vi "xy_bar_graph.vi"() -> ()   [LabVIEW 2016]
doc: "This VI demonstrates how to create a bar graph in LabVIEW by plotting data to an XY graph. This VI converts the data that appears in a table to bars and groups the bars by column of data from the table."
panel:
  out "Annual Report":cluster{dbl[], dbl[]}[](graph)
  in  "Table":string[][](table)=[["34", "74", "23", "35", "23", "26", "74", "74", "21", "39", "61", "83"], ["73", "24", "75", "87", "42", "34", "35", "76", "52", "43", "43", "3"], ["36", "25", "12", "34", "24", "74", "73", "54", "88", "64", "90", "62"]]
  # "This VI graphs the data from the Table to the Annual Report graph.  Select Help»Show Context Help and move the cursor over the VI icon to display help for this VI."
  # "Jan"
  # "Feb"
  # "Mar"
  # "April"
  # "May"
  # "June"
  # "July"
  # "Aug"
  # "Sept"
  # "Oct"
  # "Nov"
  # "Dec"
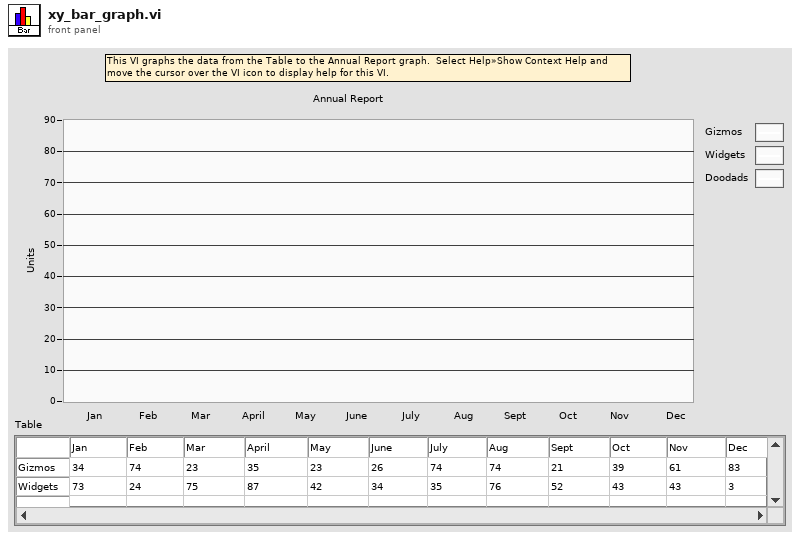
[diagram p1: front panel]
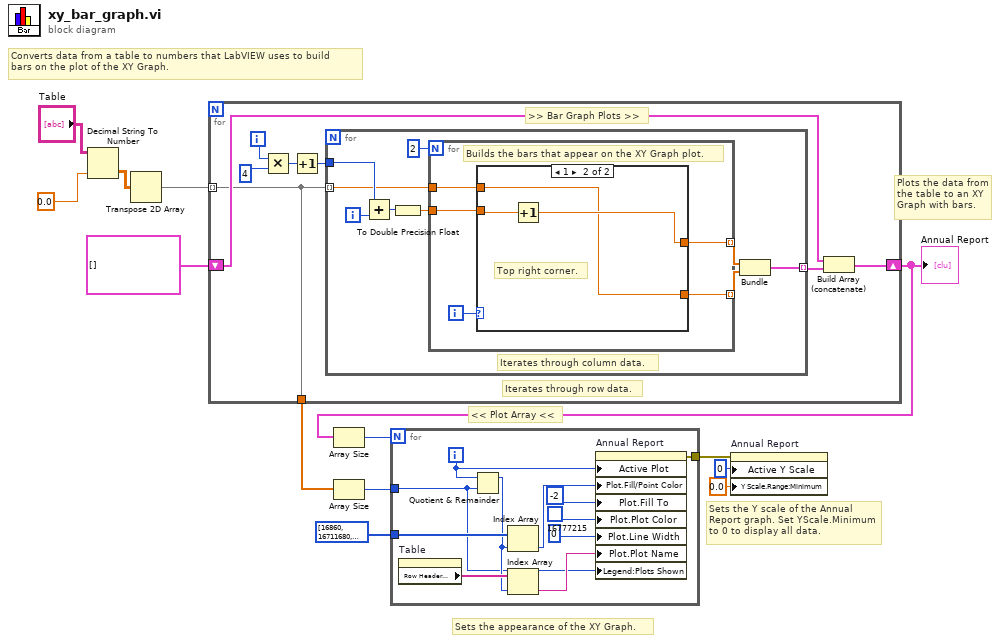
[diagram p0: block diagram]
diagram:
  # "Plots the data from the table to an XY Graph with bars."
  # "Converts data from a table to numbers that LabVIEW uses to build \nbars on the plot of the XY Graph."
  # "Sets the appearance of the XY Graph."
  # "Sets the Y scale of the Annual Report graph. Set YScale.Minimum to 0 to display all data."
  # "<< Plot Array <<"
  n1 = Decimal String To Number(string="Table", default (0L)=0.0) -> (number=w11:dbl[][])  [unwired: 1 in, 1 out]
  n2 = Transpose 2D Array(2D array=w11) -> (transposed array=w10:dbl[][])
  n3 = for {
    tunnel: w10 -> [w14] mode=indexing
    shift-right: [w18] -> w8
    shift-left: cluster{dbl[], dbl[]}[] [] -> [w17]
    tunnel: [w14] -> w6
    i -> [w21]
    # "Iterates through row data."
    # ">> Bar Graph Plots >>"
    n4 = Multiply(x=w21, y=4) -> (x*y=w16:i32)
    n5 = Increment(x=w16) -> (x+1=w15:i32)
    n6 = for {
      tunnel: w14 -> [w23] mode=indexing
      tunnel: w15 -> [w30]
      tunnel: [w25] -> w19 mode=indexing
      i -> [w24]
      # "Iterates through column data."
      n7 = Add(x=w30, y=w24) -> (x+y=w29:i32)
      n8 = To Double Precision Float(number=w29) -> (double precision float=w28:dbl)
      n9 = for {
        N: 2 -> [_]
        tunnel: w23 -> [w34]
        tunnel: [w33] -> w26 mode=indexing
        tunnel: w28 -> [w32]
        tunnel: [w31] -> w27 mode=indexing
        i -> [w35]
        # "Builds the bars that appear on the XY Graph plot."
        n10 = case shown="1" w35 {
          tunnel: w34 -> [w37 w38]
          tunnel: [w37 w38] -> w33
          tunnel: w32 -> [w36 w40]
          tunnel: [w36 w39] -> w31
          frame 0, Default {
            # "Top left corner."
          }
          frame 1 {
            # "Top right corner."
            n11 = Increment(x=w40) -> (x+1=w39:dbl)
          }
        }
      }
      n12 = Bundle(w27, w26) -> (w25:cluster{dbl[], dbl[]})  [unwired: 1 in]
    }
    n13 = Build Array (concatenate) "Build Array"(w17, w19) -> (w18:cluster{dbl[], dbl[]}[])
  }
  "Annual Report" <- w8
  n14 = Array Size(array=w8) -> (size(s)=w7:i32)
  n15 = Array Size(array=w6) -> (size(s)=w5:i32)
  n16 = for {
    N: w7 -> [_]
    tunnel: w5 -> [w42]
    tunnel: u32[] [16860, 16711680, 1175296, 16773632, 15679744, 16711925, 2818015, 4325415] -> [w47]
    tunnel: [w41] -> w3
    i -> [w51]
    n17 = property on="Table" class="Tbl (strict)"() -> ("Row Header Strings[]"=w45:string[])  [unwired: 2 in, 2 out]
    n18 = Quotient & Remainder(x=w51, y=w42) -> (x-y*floor(x/y)=w44:i32)  [unwired: 1 out]
    n19 = Index Array(array=w47, index=w44) -> (element=w50:u32)
    n20 = Index Array(array=w45, index=w44) -> (element=w43:string)
    n21 = property on="Annual Report" class="XYGraph (strict)"("Active Plot"=w51, "Plot.Fill/Point Color"=w50, "Plot.Fill To"=i16 -2, "Plot.Plot Color"=u32 16777215, "Plot.Line Width"=u8 0, "Plot.Plot Name"=w43, "Legend:Plots Shown"=w42) -> (error out=w41:errorcluster)  [unwired: 2 in, 1 out]
  }
  n22 = property on="Annual Report" class="XYGraph (strict)"(error in=w3, "Active Y Scale"=0 ("Active X Scale"), "Y Scale.Range:Minimum"=0.0 ("X Scale.Range:Maximum")) -> ()  [unwired: 1 in, 2 out]
